vi "Exercise 5-2 Main.vi"(2 "Error In":errorcluster, 3 "Weather Data In":T1={"Current Temperature"=0.0, "Max Temperature"=0.0, "Min Temperature"=0.0, "Warning?"=FALSE, "Warning Text"="No Warning", "Units"=0} {"Units" items=["Celsius", "Fahrenheit"]}) -> (0 "Error Out":errorcluster, 1 "Weather Data Out":T1={"Current Temperature"=0.0, "Max Temperature"=0.0, "Min Temperature"=0.0, "Warning?"=FALSE, "Warning Text"="No Warning", "Units"=0} {"Units" items=["Celsius", "Fahrenheit"]})   [LabVIEW 2015]
uses:
  Exercise 5-2 Weather Data.ctl
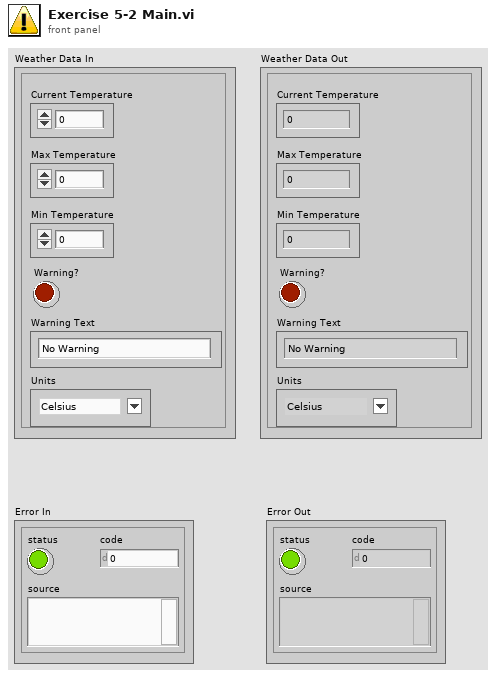
[diagram p1: front panel]
types:
  T1 = typedef "Exercise 5-2 Weather Data.ctl" = cluster{"Current Temperature":dbl, "Max Temperature":dbl, "Min Temperature":dbl, "Warning?":bool, "Warning Text":string, "Units":u16}
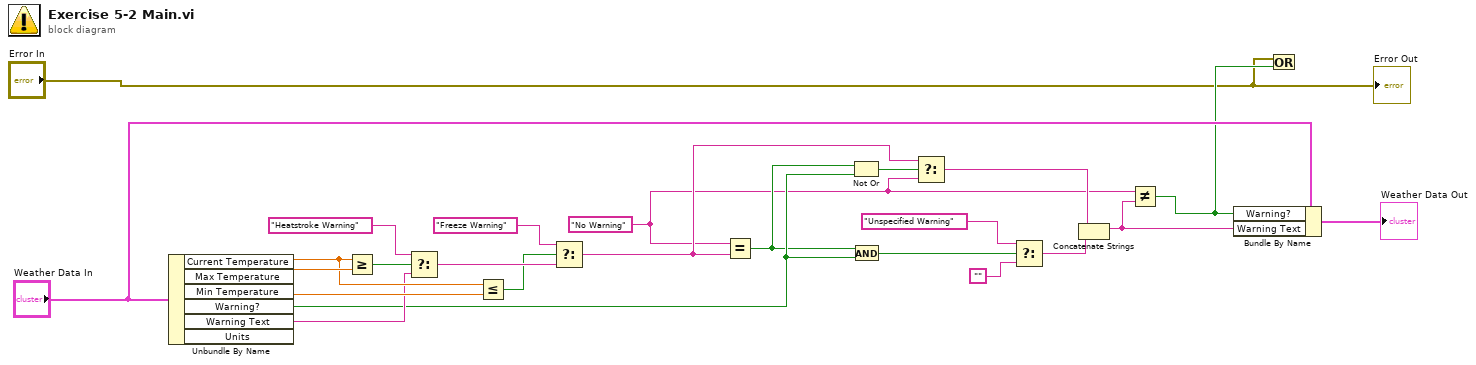
[diagram p0: block diagram]
diagram:
  w4 = "No Warning"
  n1 = Unbundle By Name("Weather Data In") -> ("Current Temperature"=w21:dbl, "Max Temperature"=w24:dbl, "Min Temperature"=w20:dbl, "Warning?"=w13:bool, "Warning Text"=w14:string)  [unwired: 1 out]
  n2 = Greater Or Equal?(x=w21, y=w24) -> (x >= y?=w23:bool)
  n3 = Select(t="Heatstroke Warning", s=w23, f=w14) -> (s? t:f=w18:string)
  n4 = Less Or Equal?(x=w21, y=w20) -> (x <= y?=w17:bool)
  n5 = Select(t="Freeze Warning", s=w17, f=w18) -> (s? t:f=w10:string)
  n6 = Equal?(x=w4, y=w10) -> (x = y?=w12:bool)
  n7 = Not Or(1:w13, 2:w12) -> (0:w11:bool)
  n8 = And(x=w12, y=w13) -> (x .and. y?=w16:bool)
  n9 = Select(t=w10, s=w11, f=w4) -> (s? t:f=w8:string)
  n10 = Select(t="Unspecified Warning", s=w16, f="") -> (s? t:f=w7:string)
  n11 = Concatenate Strings(w8, w7) -> (w3:string)
  n12 = Not Equal?(x=w4, y=w3) -> (x != y?=w2:bool)
  n13 = Bundle By Name(cluster="Weather Data In", "Warning?"=w2, "Warning Text"=w3) -> (→"Weather Data Out":T1)
  n14 = Or(x="Error In", y=w2) -> ()  [unwired: 1 out]
  "Error Out" <- "Error In"
